vi "Send_Balance.vi"(8 "error in (no error)":errorcluster, 11 "Balance_check in":refnum<class "Balance_check.lvclass">) -> (0 "error out":errorcluster, 3 "Balance_check out":refnum<class "Balance_check.lvclass">)   [LabVIEW 2025, in "User_Console.lvlib" / "Balance_check.lvclass"]
uses:
  Balance_check.lvclass
  Balance_check.lvclass/Balance_check.ctl
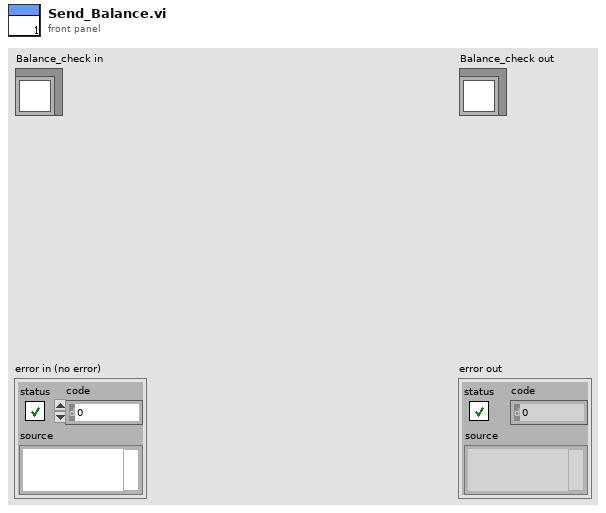
[diagram p1: front panel]
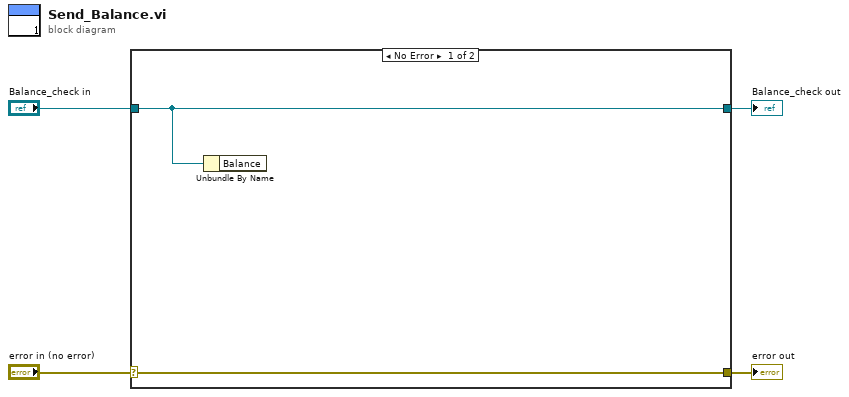
[diagram p0: block diagram]
diagram:
  n1 = case shown="No Error" "error in (no error)" {
    selector: "error in (no error)" -> [w6 w8]
    tunnel: [w6 w8] -> w3
    tunnel: [w5 w7] -> w1
    tunnel: "Balance_check in" -> [w5 w7]
    frame No Error {
      n2 = Unbundle By Name(w5) -> ()  [unwired: 1 out]
    }
    frame Error {
    }
  }
  "error out" <- w3
  "Balance_check out" <- w1
